vi "accuvim(SubVI).vi"(10 "stop":bool, 11 "VISA Refnum in":refnum<visa-resource-name>="COM7") -> (1 "Current (A)":dbl, 2 "Voltage (V)":dbl, 3 "frequncy (Hz)":sgl, 4 "Power (W)":dbl)   [LabVIEW 2012]
uses:
  <vilib>/Instr/_visa.llb/VISA Configure Serial Port (Instr).vi
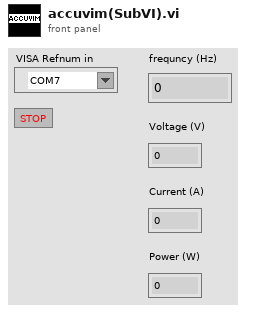
[diagram p1: front panel]
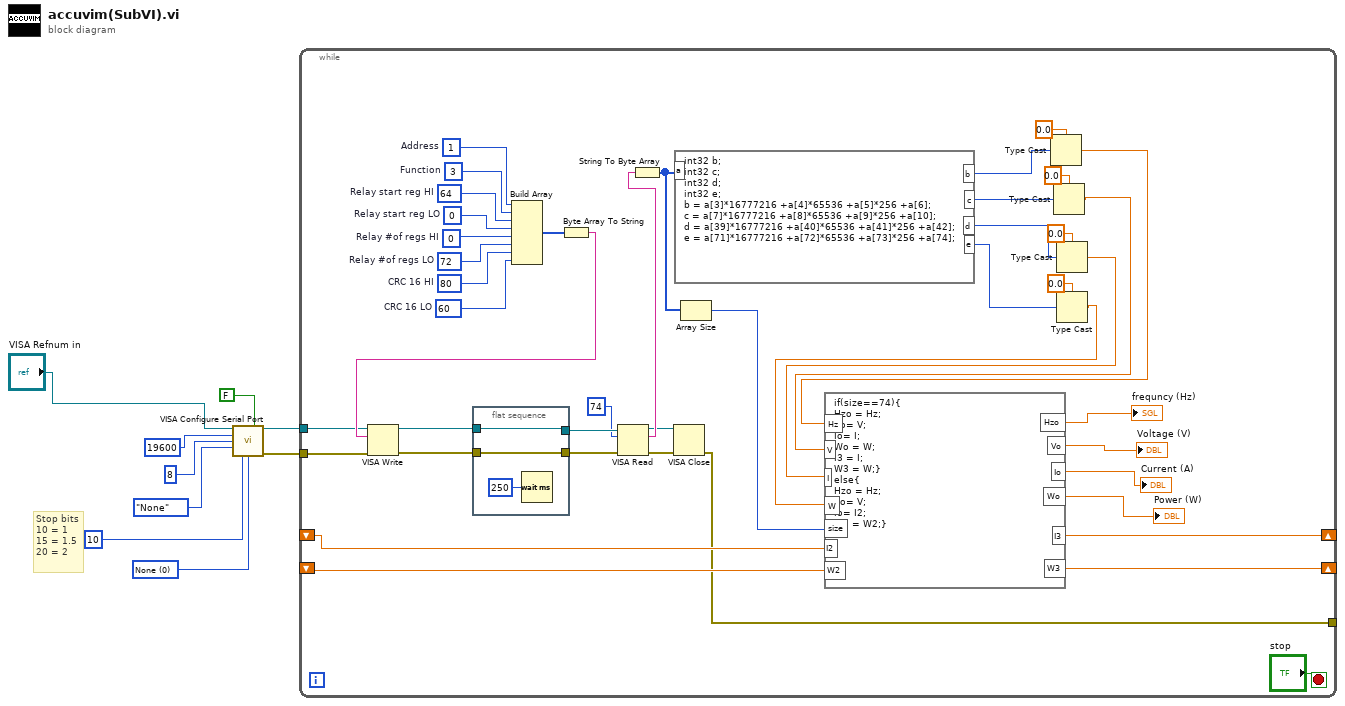
[diagram p0: block diagram]
diagram:
  w5 = u16 0 items=["None", "XON/XOFF", "RTS/CTS", "XON/XOFF & RTS/CTS", "DTR/DSR", "XON/XOFF & DTR/DSR"] ("flow control (0:none)")
  # "Stop bits\n10 = 1\n15 = 1.5\n20 = 2"
  n1 = call-poly "VISA Configure Serial Port"("VISA resource name"="VISA Refnum in", "Enable Termination\nChar (T)"=FALSE ("Enable Termination\nChar (T)"), "baud rate (9600)"=u32 19600, "data bits (8)"=u16 8, "parity (0:none)"=enum16{"None", "Odd", "Even", "Mark", "Space"}."None", "stop bits (10: 1 bit)"=10, "flow control (0:none)"=w5) -> ("VISA resource name out"=w8:refnum<visa-resource-name>, "error out"=w9:errorcluster)  [unwired: 7 in]
  n2 = while {
    shift-right: [w19] -> _
    shift-left: _ -> [w17]
    shift-right: [w18] -> _
    shift-left: _ -> [w16]
    tunnel: [w15] -> _
    tunnel: w8 -> [w14]
    tunnel: w9 -> [w13]
    stop <- "stop" stop-if-true
    w47 = 60  # CRC 16 LO
    w46 = 80  # CRC 16 HI
    w45 = 72  # Relay #of regs LO
    w44 = 0  # Relay #of regs HI
    w43 = 0  # Relay start reg LO
    w41 = 64  # Relay start reg HI
    w42 = 3  # Function
    w49 = 1  # Address
    n3 = flat-sequence {
      tunnel: [w55] -> w51
      tunnel: w53 -> [w55]
      tunnel: [w54] -> w50
      tunnel: w52 -> [w54]
      frame #0 {
        n4 = Wait (ms)(milliseconds to wait=u32 250) -> ()  [unwired: 1 out]
      }
    }
    n5 = Build Array(w49, w42, w41, w43, w44, w45, w46, w47) -> (w48:i32[])
    n6 = Byte Array To String(unsigned byte array=w48) -> (string=w40:string)
    n7 = VISA Write(VISA resource name=w14, write buffer=w40, error in (no error)=w13) -> (VISA resource name out=w53:refnum<visa-resource-name>, error out=w52:errorcluster)  [unwired: 1 out]
    n8 = VISA Read(VISA resource name=w51, byte count=u32 74, error in (no error)=w50) -> (VISA resource name out=w23:refnum<visa-resource-name>, read buffer=w31:string, error out=w22:errorcluster)  [unwired: 1 out]
    n9 = String To Byte Array(string=w31) -> (unsigned byte array=w25:u8[])
    n10 = VISA Close(VISA resource name=w23, error in (no error)=w22) -> (error out=w15:errorcluster)
    n11 = formula code="int32 b;\nint32 c;\nint32 d;\nint32 e;\nb = a[3]*16777216 +a[4]*65536 +a[5]*256 +a[6];\nc = a[7]*16777216 +a[8]*65536 +a[9]*256 +a[10];\nd = a[39]*16777216 +a[40]*65536 +a[41]*256 +a[42];\ne = a[71]*16777216 +a[72]*65536 +a[73]*256 +a[74];"("a"=w25) -> ("b"=w34:i32, "c"=w36:i32, "e"=w38:i32, "d"=w30:i32)
    n12 = Array Size(array=w25) -> (size(s)=w24:i32)
    n13 = Type Cast(type=sgl 0.0, x=w34) -> (*(type *) &x=w29:sgl)
    n14 = Type Cast(type=sgl 0.0, x=w36) -> (*(type *) &x=w28:sgl)
    n15 = Type Cast(type=sgl 0.0, x=w30) -> (*(type *) &x=w27:sgl)
    n16 = Type Cast(type=sgl 0.0, x=w38) -> (*(type *) &x=w26:sgl)
    n17 = formula code="if(size==74){\nHzo = Hz;\nVo= V;\nIo= I;\nWo = W;\nI3 = I;\nW3 = W;}\nelse{\nHzo = Hz;\nVo= V;\nIo= I2;\nWo = W2;}"("Hz"=w29, "V"=w28, "I"=w27, "W"=w26, "I2"=w17, "W2"=w16, "size"=w24) -> ("Hzo"=→"frequncy (Hz)":dbl, "Vo"=→"Voltage (V)":dbl, "Io"=→"Current (A)":dbl, "Wo"=→"Power (W)":dbl, "I3"=w19:dbl, "W3"=w18:dbl)
  }
